vi "Signal_Hound_Live_Sweeping.vi"(0 "error in (no error)":errorcluster, 1 "device":i32) -> ()   [LabVIEW 2024]
doc: "Continuously acquire sweep data from a Signal Hound SA Series Spectrum Analyzer."
uses:
  <vilib>/Utility/xml.llb/Read From XML File(string).vi
  <vilib>/Utility/xml.llb/Write to XML File(string).vi
  <instrlib>/Signal Hound SA Series/Signal Hound SA Series.lvlib
panel:
  out "Peak Frequency (Hz)":sgl format="%^#.4g"
  out "Peak Amplitude (dBm)":sgl format="%#.2g"
  in  "VBW (Hz)":dbl=30000.0 format="%^#.4g"
  in  "RBW (Hz)":dbl=30000.0 format="%^#.4g"
  out "error out":errorcluster
  in  "Reject":bool=TRUE
  in  "Flag":i32 caption="Status"
  in  "Mode":i32 caption="Status"
  out "Start Frequency (Hz)":dbl format="%^#.4g"
  out "Bin Size (Hz)":dbl format="%^#.4g"
  in  "?":bool
  out "min output":dbl[](array[numeric]) caption="Min"
  out "max output":dbl[](array[numeric]) caption="Max"
  in  "Ref Level (dBm)":dbl=-30.0 format="%^#.2g"
  out "Waveform Graph":T1(graph)
  in  "Span (Hz)":dbl=100000000.0 format="%^#.4g"
  in  "Center Frequency (Hz)":dbl=1000000000.0 min=1.0 max=4400000000.0 step=1.0 format="%^#.4g"
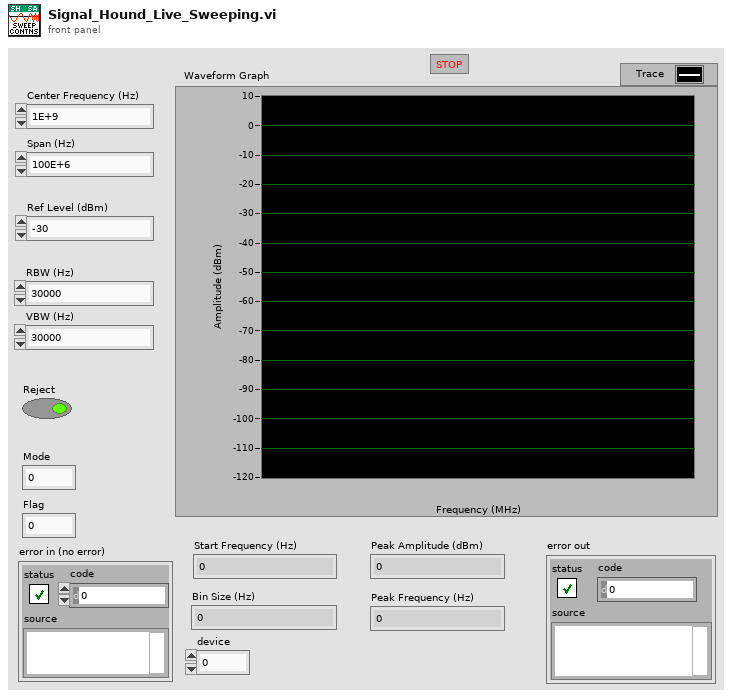
[diagram p1: front panel]
types:
  T1 = cluster{"startFreq out":dbl, "binSize out":dbl, "max out":sgl[]}
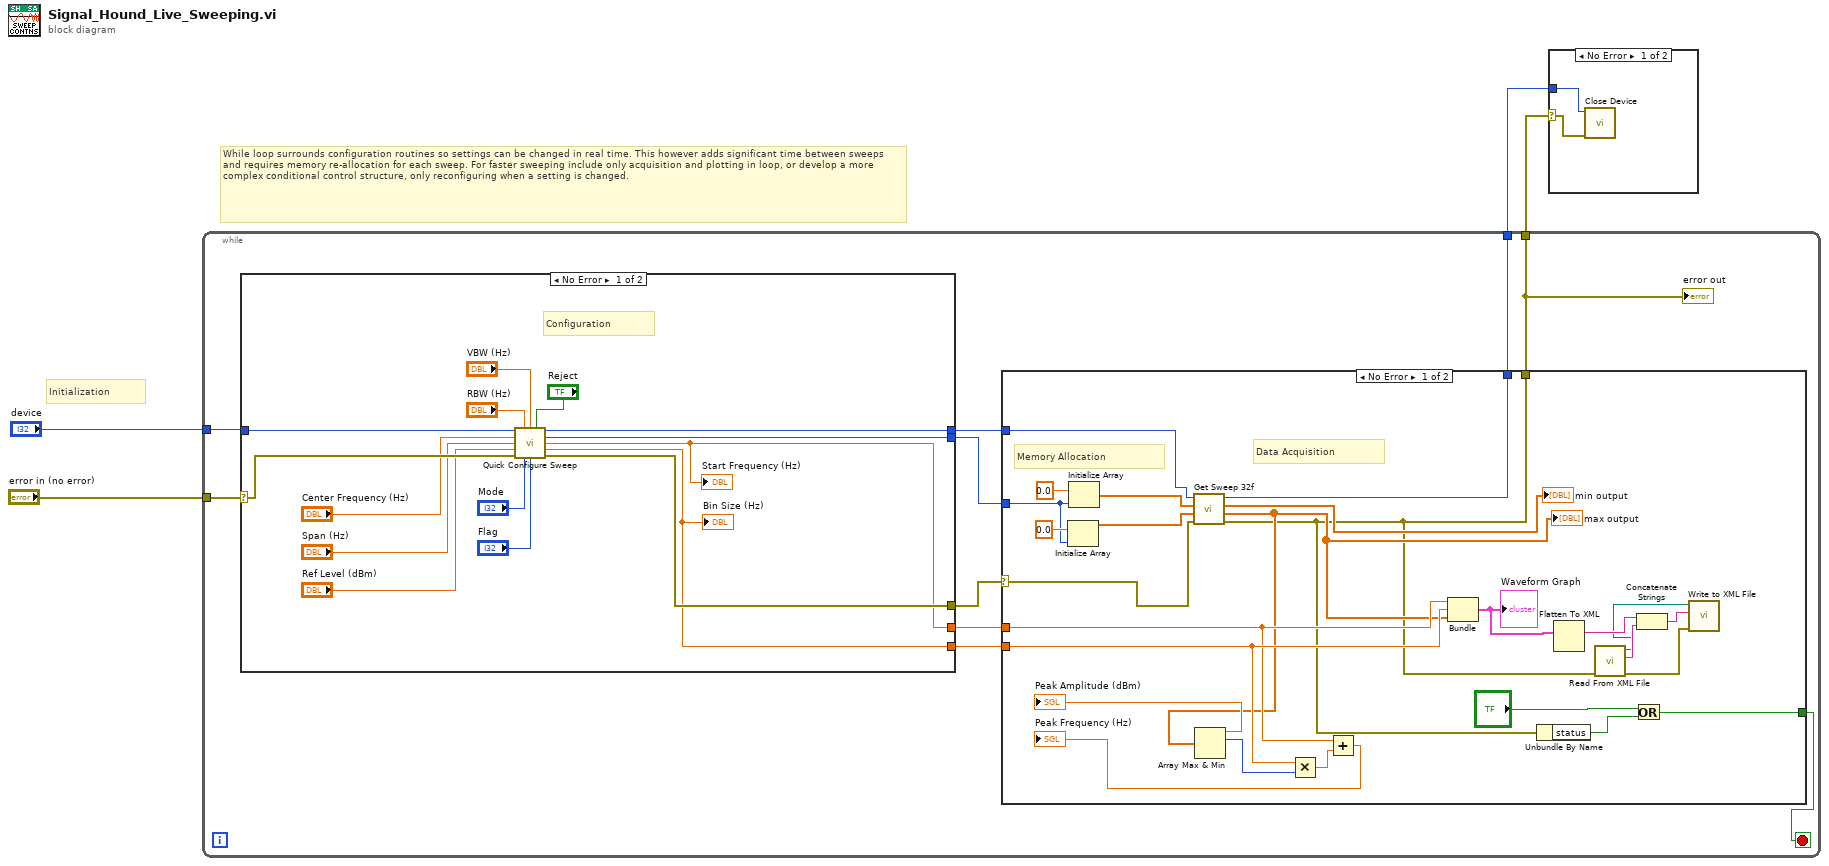
[diagram p0: block diagram]
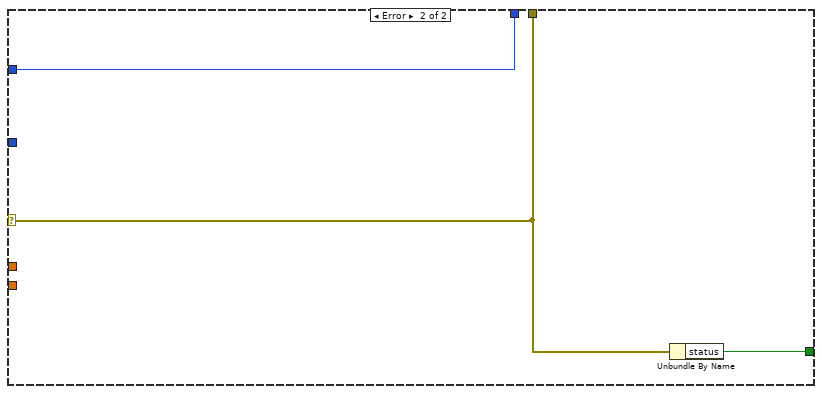
[diagram p2: hidden frame]
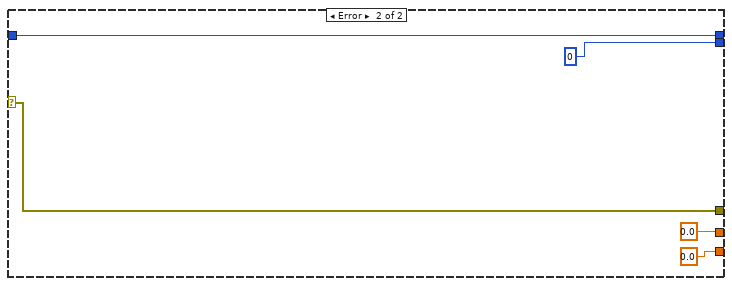
[diagram p3: hidden frame]
diagram:
  # "While loop surrounds configuration routines so settings can be changed in real time. This however adds significant time between sweeps and requires memory re-allocation for each sweep. For faster sweeping include only acquisition and plotting in loop, or develop a more complex conditional control structure, only reconfiguring when a setting is changed."
  # "Initialization"
  n1 = while {
    tunnel: [w8] -> w4
    tunnel: [w5] -> w3
    tunnel: "device" -> [w7]
    tunnel: "error in (no error)" -> [w6]
    stop <- w9 stop-if-true
    n2 = case shown="No Error" w6 {
      selector: w6 -> [w52 w63]
      tunnel: w7 -> [w57 w62]
      tunnel: [w55 w62] -> w14
      tunnel: [w54 w63] -> w12
      tunnel: [w53 0] -> w13
      tunnel: [w44 0.0] -> w11
      tunnel: [w51 0.0] -> w10
      frame No Error {
        # "Configuration"
        n3 = call <instrlib>:"Quick Configure Sweep.vi"("device"=w57, "rbw"="RBW (Hz)", "vbw"="VBW (Hz)", "reject"="Reject", "center"="Center Frequency (Hz)", "span"="Span (Hz)", "ref"="Ref Level (dBm)", "error in"=w52, "mode"="Mode", "flag"="Flag") -> ("device out"=w55:i32, "sweepLength out"=w53:i32, "startFreq out"=w44:dbl, "binSize out"=w51:dbl, "error out"=w54:errorcluster)  [unwired: 1 in]
        "Bin Size (Hz)" <- w51
        "Start Frequency (Hz)" <- w44
      }
      frame Error {
      }
    }
    n4 = case shown="No Error" w12 {
      selector: w12 -> [w33 w42]
      tunnel: [w40 w43] -> w8
      tunnel: w14 -> [w35 w43]
      tunnel: w13 -> [w34 _]
      tunnel: [w18 w42] -> w5
      tunnel: w11 -> [w24 _]
      tunnel: w10 -> [w25 _]
      tunnel: [w29 w41] -> w9
      frame No Error {
        # "Data Acquisition"
        # "Memory Allocation"
        n5 = Initialize Array(sgl 0.0, w34) -> (w36:sgl[])
        n6 = Initialize Array(sgl 0.0, w34) -> (w37:sgl[])
        n7 = call <instrlib>:"Get Sweep 32f.vi"("error in (no error)"=w33, "max"=w36, "min"=w37, "device"=w35) -> ("error out"=w18:errorcluster, "max out"=w23:sgl[], "min out"=→"min output":sgl[], "device out"=w40:i32)  [unwired: 4 in]
        "max output" <- w23
        n8 = Array Max & Min(array=w23) -> (max value=→"Peak Amplitude (dBm)":sgl, max index (indices)=w28:i32)  [unwired: 2 out]
        n9 = Multiply(x=w25, y=w28) -> (x*y=w26:dbl)
        n10 = Add(x=w24, y=w26) -> (x+y=→"Peak Frequency (Hz)":dbl)
        n11 = Bundle("startFreq out"=w24, "binSize out"=w25, "max out"=w23) -> (w16:T1)  [unwired: 1 in]
        "Waveform Graph" <- w16
        n12 = Unbundle By Name(w18) -> ("status"=w30:bool)
        n13 = Flatten To XML(6:w16) -> (2:w17:string)
        n14 = call-poly <vilib>:"Read From XML File.vi"("error in (no error)"=w18) -> ("error out"=w19:errorcluster, "XML Elements"=w21:string, "XML File Path(duplicate)"=w15:path)  [unwired: 8 in]
        n15 = Or(x="?", y=w30) -> (x .or. y?=w29:bool)
        n16 = Concatenate Strings(w17, w21) -> (w20:string)
        n17 = call-poly <vilib>:"Write to XML File.vi"("error in (no error)"=w19, "XML Input"=w20, "XML File Path"=w15) -> ()  [unwired: 6 in, 3 out]
      }
      frame Error {
        n18 = Unbundle By Name(w42) -> ("status"=w41:bool)
      }
    }
    "error out" <- w5
  }
  n19 = case shown="No Error" w3 {
    selector: w3 -> [w64 _]
    tunnel: w4 -> [w65 _]
    frame No Error {
      n20 = call <instrlib>:"Close Device.vi"("error in (no error)"=w64, "device"=w65) -> ()  [unwired: 8 in, 2 out]
    }
    frame Error {
    }
  }
